vi "Add Offset to Waveform.vi"(0 "signal configuration":refnum<class "SV Signal.lvclass">, 5 "input waveform":waveform(dbl), 11 "error in (no error)":errorcluster) -> (4 "signal configuration":refnum<class "SV Signal.lvclass">, 6 "offset waveform":waveform(dbl), 10 "DCOffset":dbl, 15 "error out":errorcluster)   [LabVIEW 2017, in "SV Signal.lvclass"]
uses:
  <vilib>/addons/_NISVFA/_Generation/Signal Generation/SV Signal/SV Signal.lvclass
  <vilib>/addons/_NISVFA/_Generation/Signal Generation/SV Signal/SV Signal.lvclass/SV Signal.ctl
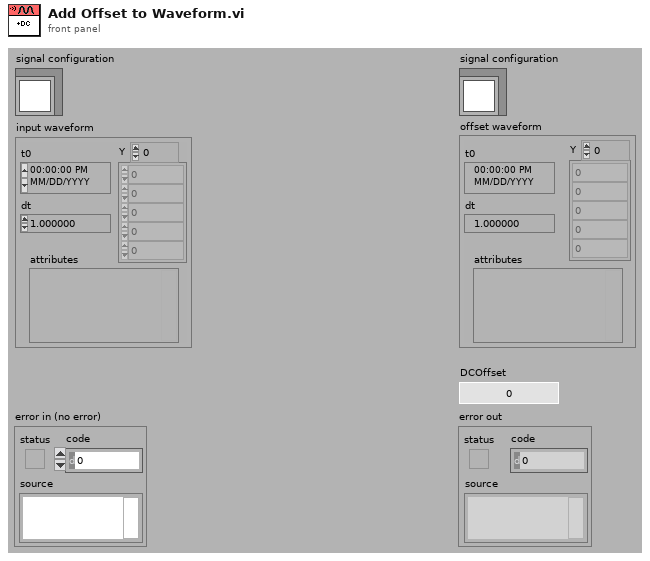
[diagram p1: front panel]
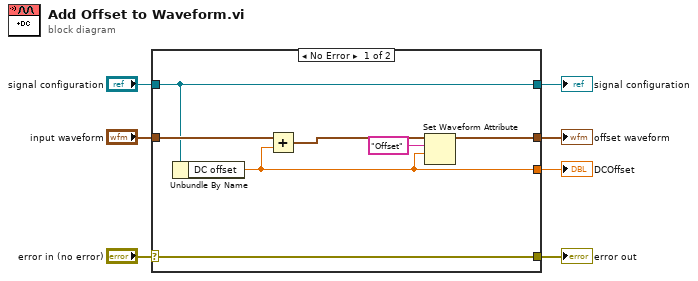
[diagram p0: block diagram]
diagram:
  n1 = case shown="No Error" "error in (no error)" {
    selector: "error in (no error)" -> [w14 w16]
    tunnel: [w14 w16] -> w6
    tunnel: [w8 w17] -> w4
    tunnel: "signal configuration" -> [w8 w17]
    tunnel: [w9 _] -> w3
    tunnel: "input waveform" -> [w13 w15]
    tunnel: [w11 w15] -> w1
    frame No Error {
      n2 = Unbundle By Name(w8) -> ("DC offset"=w9:dbl)
      n3 = Add(x=w13, y=w9) -> (x+y=w12:waveform(dbl))
      n4 = Set Waveform Attribute(5:w9, 6:"Offset" ("name"), 7:w12) -> (3:w11:waveform(dbl))  [unwired: 1 in, 2 out]
    }
    frame Error {
    }
  }
  "error out" <- w6
  "signal configuration" <- w4
  "DCOffset" <- w3
  "offset waveform" <- w1
